vi "set_ai_noise_filter.vi"(8 "error in (no error)":errorcluster, 10 "Line frequency":enum16{"60 Hz", "50 Hz"}(ring), 11 "Modbus Master in":refnum<class "Modbus Master.lvclass">) -> (0 "error out":errorcluster, 3 "Modbus Master out":refnum<class "Modbus Master.lvclass">)   [LabVIEW 2018]
uses:
  <vilib>/NI/Modbus Library/API/Master/Modbus Master.lvclass
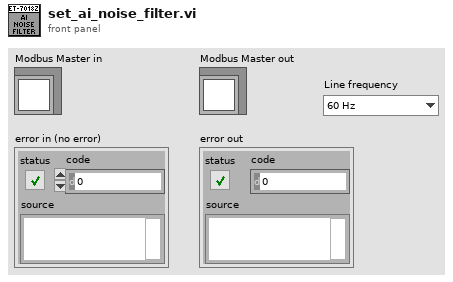
[diagram p1: front panel]
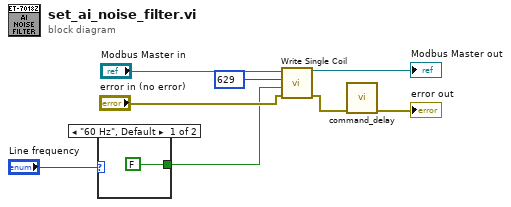
[diagram p0: block diagram]
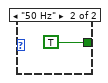
[diagram p2: hidden frame]
diagram:
  n1 = case shown="\"60 Hz\", Default" "Line frequency" {
    tunnel: [FALSE TRUE] -> w3
    frame "60 Hz", Default {
    }
    frame "50 Hz" {
    }
  }
  n2 = call-dynamic "Write Single Coil.vi"("error in"="error in (no error)", "coil to write"=w3, "address"=u16 629 ("starting address"), "Modbus master in"="Modbus Master in") -> ("error out"=w2:errorcluster, "Modbus master out"=→"Modbus Master out":refnum<class "Modbus Master.lvclass">)  [unwired: 6 in]
  n3 = call "command_delay.vi"("error in (no error)"=w2) -> ("error out"=→"error out":errorcluster)  [unwired: 10 in]
